vi "PH_ImageCalibrator.allocate or free img space.vi"(0 "i ref in":refnum<vi>, 2 "Allocate?":bool, 5 "error in (no error)":errorcluster) -> (14 "i ref out":refnum<vi>, 19 "error out":errorcluster)   [LabVIEW 2014, in "PH_ImageCalibrator.lvlib"]
doc: "This VI is forseen to be used in constructor or destructor. If Allocate? = true is chosen, memory space for several images is allocated. If false is chosen, it is freed."
uses:
  PH_ImageCalibrator.lvlib
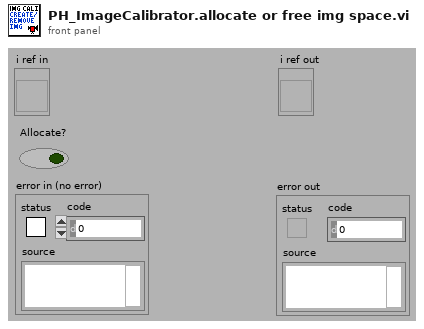
[diagram p1: front panel]
types:
  T1 = typedef "PH_ImageCalibrator.lvlib/PH_ImageCalibrator.i attribute.ctl" = cluster{"GUI Refs":cluster{"Available Cams":refnum<vi>, "OK":refnum<vi>, "Skip":refnum<vi>, "Repeat":refnum<vi>, "Cancel":refnum<vi>, "Length [mm]":refnum<vi>, "Energy [mJ]":refnum<vi>, "Dialog":refnum<vi>}, "Cam instances":string[], "Dark Pics":cluster{"#":i32, "BI taken":bool}, "Lin Cali":cluster{"Distance [Pixel]":dbl, "Distance [mm]":dbl, "Lin Cali Factor [mm/Pixel]":dbl}, "Energy Cali":cluster{"Pixelsum":dbl, "Energy [mJ]":dbl, "Energy Cali factor [mJ/Pixelsum]":dbl, "Underground subtracted?":bool, "#":i32}, "Images":cluster{"Background":T2, "Energy":T2}}
  T2 = typedef "IMAQ Image.ctl" = refnum<image>
  T3 = typedef "Image Type" = u32
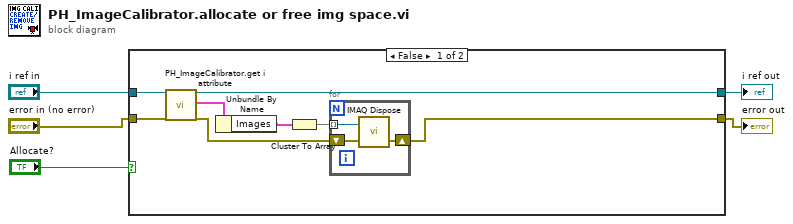
[diagram p0: block diagram]
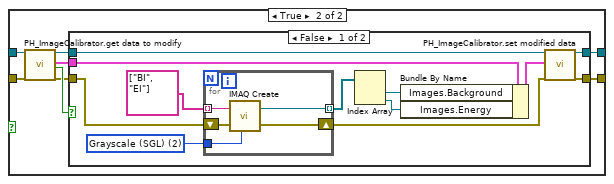
[diagram p2: hidden frame]
diagram:
  n1 = case shown="False" "Allocate?" {
    tunnel: [w8 w23] -> w5
    tunnel: [w10 w22] -> w4
    tunnel: "error in (no error)" -> [w13 w19]
    tunnel: "i ref in" -> [w12 w18]
    frame False {
      n2 = call "PH_ImageCalibrator.get i attribute.vi"("i ref in"=w12, "error in (no error)"=w13) -> ("i ref out"=w10:refnum<vi>, "i attribute"=w11:T1, "error out"=w9:errorcluster)  [unwired: 15 in]
      n3 = Unbundle By Name(w11) -> ("Images"=w7:cluster{"Background":T2, "Energy":T2})
      n4 = Cluster To Array(cluster=w7) -> (array=w6:T2[])
      n5 = for {
        shift-right: [w15] -> w8
        shift-left: w9 -> [w16]
        tunnel: w6 -> [w14] mode=indexing
        n6 = call "IMAQ Dispose"("Image"=w14, "error in (no error)"=w16) -> ("error out"=w15:errorcluster)  [unwired: 4 in]
      }
    }
    frame True {
      n7 = call "PH_ImageCalibrator.get data to modify.vi"("i ref in"=w18, "error in (no error)"=w19) -> ("i ref out"=w21:refnum<vi>, "i attribute"=w17:T1, "timed out"=w24:bool, "error out"=w20:errorcluster)  [unwired: 14 in]
      n8 = case shown="False" w24 {
        tunnel: w20 -> [w30 w42]
        tunnel: w21 -> [w36 w43]
        tunnel: [w35 w43] -> w22
        tunnel: [w34 w42] -> w23
        tunnel: w17 -> [w33 _]
        frame False {
          w25 = T3 2 items=["Grayscale (U8)", "Grayscale (I16)", "Grayscale (SGL)", "Complex (CSG)", "RGB (U32)", "HSL (U32)", "RGB (U64)"] ("Image Type")
          n9 = for {
            shift-right: [w41] -> w31
            shift-left: w30 -> [w40]
            tunnel: [w37] -> w29 mode=indexing
            tunnel: string[] ["BI", "EI"] -> [w39] mode=indexing
            tunnel: w25 -> [w38]
            n10 = call "IMAQ Create"("Image Name"=w39, "Image Type"=w38, "error in (no error)"=w40) -> ("New Image"=w37:T2, "error out"=w41:errorcluster)  [unwired: 2 in]
          }
          n11 = Index Array(array=w29) -> (element #1=w27:T2, element #2=w26:T2)  [unwired: 2 in]
          n12 = Bundle By Name(cluster=w33, "Images.Background"=w27, "Images.Energy"=w26) -> (w32:T1)
          n13 = call "PH_ImageCalibrator.set modified data.vi"("i ref in"=w36, "i attribute"=w32, "error in (no error)"=w31) -> ("i ref out"=w35:refnum<vi>, "error out"=w34:errorcluster)  [unwired: 15 in]
        }
        frame True {
        }
      }
    }
  }
  "error out" <- w5
  "i ref out" <- w4
